vi "B_ENC (SubVI).vi"(1 "Reset Counter":bool, 7 "error in (no error)":errorcluster) -> (21 "Counter Value":i32, 22 "Counter Direction":T1, 23 "Overflow?":bool, 27 "error out":errorcluster)   [LabVIEW 2017]
doc: "Reads and decodes signals from an encoder. This Express VI reads the number of ticks that the encoder receives since the last counter reset.\n--------------------\n\nThis Express VI is configured as follows:\n\nNode name: B/Encoder\nChannel: B/ENC\nEncoder output signal type: Quadrature phase"
uses:
  <vilib>/myRIO/Common/Instrument Driver Framework/myRIO v1.0/Encoder/typedefs/Encoder Count Direction Enum.ctl
  <vilib>/myRIO/Common/Instrument Driver Framework/myRIO v1.0/Encoder/typedefs/Encoder Signal Mode.ctl
  <vilib>/myRIO/Common/Instrument Driver Framework/myRIO v1.0/Encoder/vis/myRIO v1.0 Read Encoder.vi
  <vilib>/Utility/error.llb/Error Cluster From Error Code.vi
  <vilib>/myRIO/Instrument Drivers/Onboard IO/Encoder/Encoder.lvlib
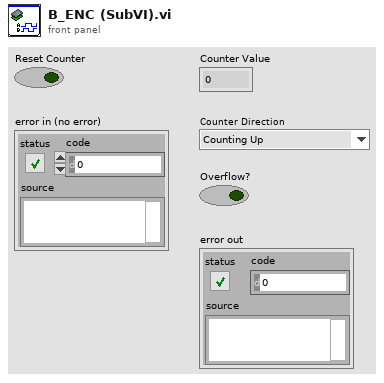
[diagram p1: front panel]
types:
  T1 = typedef "Encoder Count Direction Enum.ctl" = enum16{"Counting Up", "Counting Down"}
  T2 = typedef "Encoder Signal Mode.ctl" = enum16{"Quadrature phase signal", "Step and direction signal"}
  T3 = typedef "Encoder.lvlib/Encoder Reference.ctl" = cluster{"myRIO Reference":T4, "Encoder Channels Enum":T8}
  T4 = typedef "myRIO Generic Hardware Reference.ctl" = cluster{"myRIO Model":T5, "myRIO Hardware Reference":T6}
  T5 = typedef "Hardware Version Enum.ctl" = enum16{"Unknown", "myRIO-1900", "myRIO-1950", "roboRIO", "NI ELVIS RIO CM"}
  T6 = typedef "myRIO v1.0 Reference.ctl" = cluster{"Generic FPGA Reference":T7, "Allow multiple opens":bool}
  T7 = typedef "Generic FPGA Reference.ctl" = refnum<k20>
  T8 = typedef "Encoder Channels Enum.ctl" = enum16{"Not Connected", "C/ENC0", "C/ENC1", "A/ENC", "B/ENC", "DIO/ENC0", "DIO/ENC1", "DIO/ENC2", "DIO/ENC3", "DIO/ENC4"}
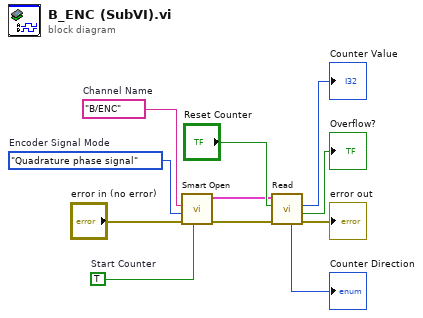
[diagram p0: block diagram]
diagram:
  w9 = TRUE  # Start Counter
  w10 = Encoder_Signal_Mode."Quadrature phase signal"  # Encoder Signal Mode
  w11 = tag "B/ENC"  # Channel Name
  n1 = call <vilib>:"Smart Open.vi"("Start Counter"=w9, "error in (no error)"="error in (no error)", "Encoder Signal Mode"=w10, "Channel Name"=w11) -> ("error out"=w2:errorcluster, "Encoder Ref Out"=w3:T3)  [unwired: 6 in]
  n2 = call <vilib>:"Read.vi"("error in (no error)"=w2, "Reset Counter"="Reset Counter", "Encoder Ref In"=w3) -> ("error out"=→"error out":errorcluster, "Overflow?"=→"Overflow?":bool, "Counter Value"=→"Counter Value":i32, "Counter Direction"=→"Counter Direction":T1)  [unwired: 4 in, 1 out]
